vi "Check Mode Delay Update.vi"(7 "TreeControl in":refnum<vi>, 8 "Analog Changed":bool=TRUE, 9 "New Num":i32, 10 "Settings In in":T1, 11 "Tree Data in":cluster{"Tag":string[], "Settings":T3[]} {"Settings"."Data Type" items=["Tree Parent"=-1, "Numeric"=0, "String"=1, "Boolean"=2, "Enum"=3]}) -> (3 "Tree Data out":cluster{"Tag":string[], "Settings":T3[]} {"Settings"."Data Type" items=["Tree Parent"=-1, "Numeric"=0, "String"=1, "Boolean"=2, "Enum"=3]})   [LabVIEW 2024, in "Sequencer with Output Values.lvlib" / "Sequencer with Output Values.lvclass"]
uses:
  Sequencer with Output Values.lvclass
  Tree Item Settings.ctl
  Data Type.ctl
  Params.ctl
  Step Settings.ctl
  Global Tree Data.vi
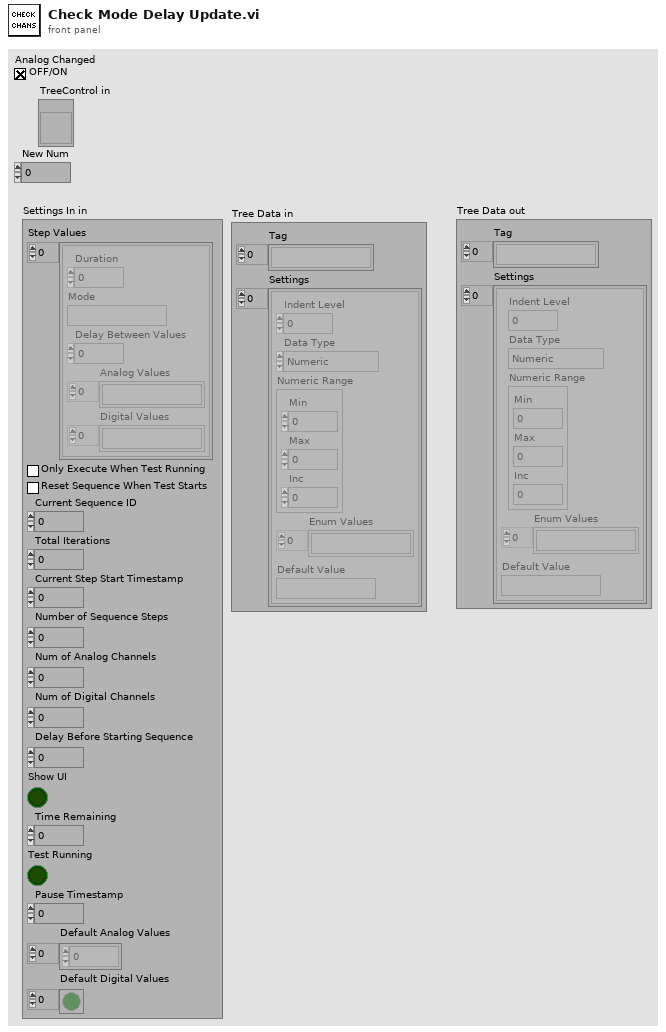
[diagram p1: front panel]
types:
  T1 = typedef "Sequencer with Output Values.lvlib/Sequencer with Output Values.lvclass/Params.ctl" = cluster{"Step Values":T2[], "Only Execute When Test Running":bool, "Reset Sequence When Test Starts":bool, "Current Sequence ID":u32, "Total Iterations":u32, "Current Step Start Timestamp":dbl, "Number of Sequence Steps":i32, "Num of Analog Channels":i32, "Num of Digital Channels":i32, "Delay Before Starting Sequence":dbl, "Show UI":bool, "Time Remaining":dbl, "Test Running":bool, "Pause Timestamp":dbl, "Default Analog Values":dbl[], "Default Digital Values":bool[]}
  T2 = typedef "Sequencer with Output Values.lvlib/Sequencer with Output Values.lvclass/Step Settings.ctl" = cluster{"Duration":dbl, "Mode":string, "Delay Between Values":dbl, "Analog Values":string[], "Digital Values":string[]}
  T3 = typedef "Sequencer with Output Values.lvlib/Sequencer with Output Values.lvclass/Tree Item Settings.ctl" = cluster{"Indent Level":i32, "Data Type":T4, "Numeric Range":cluster{"Min":dbl, "Max":dbl, "Inc":dbl}, "Enum Values":string[], "Default Value":string}
  T4 = typedef "Sequencer with Output Values.lvlib/Sequencer with Output Values.lvclass/Data Type.ctl" = i16
  T5 = cluster{"Tags Out":string[], "Settings Out":T3[]}
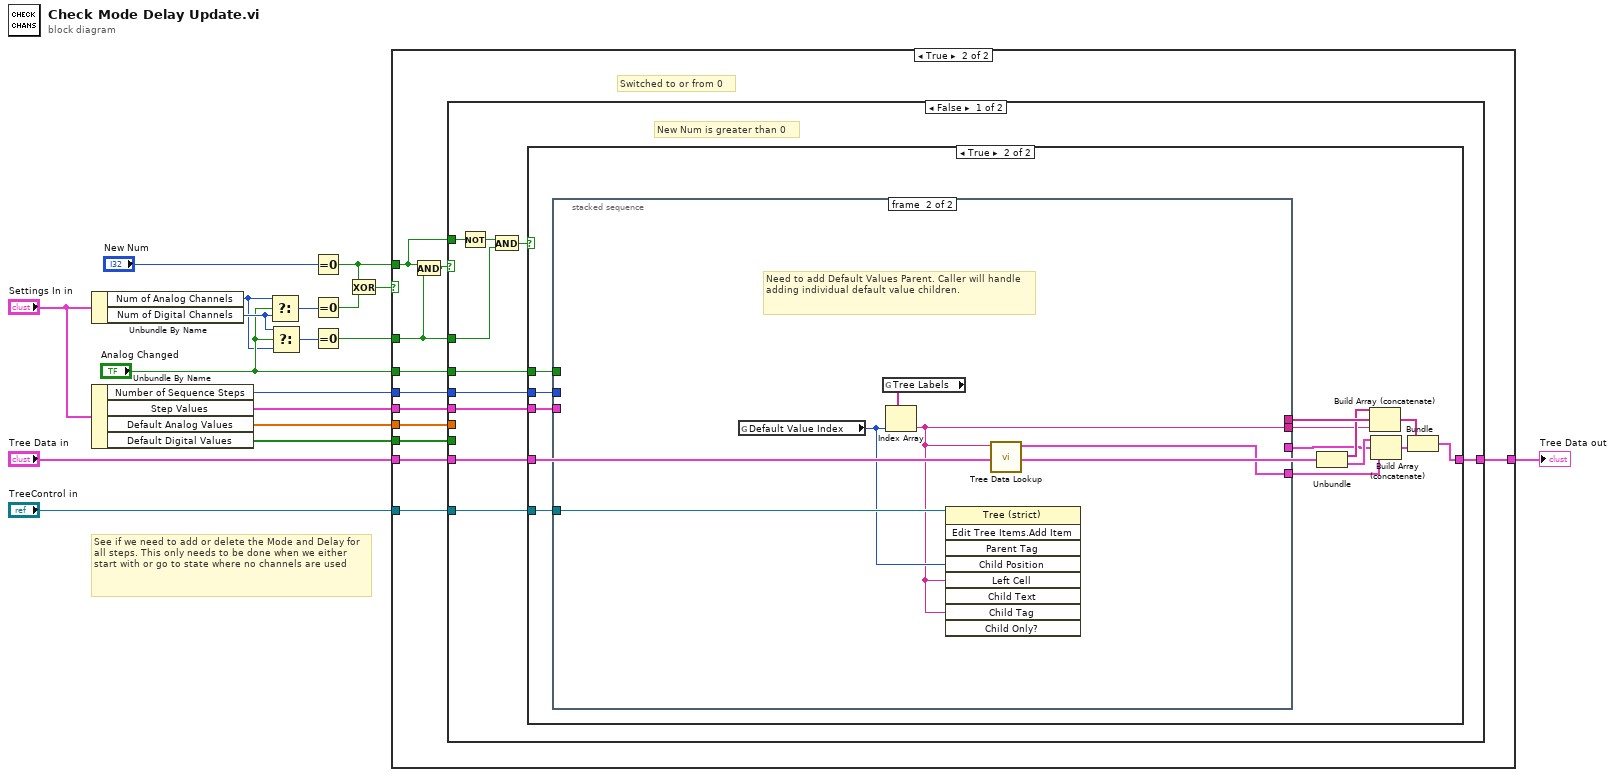
[diagram p0: block diagram]
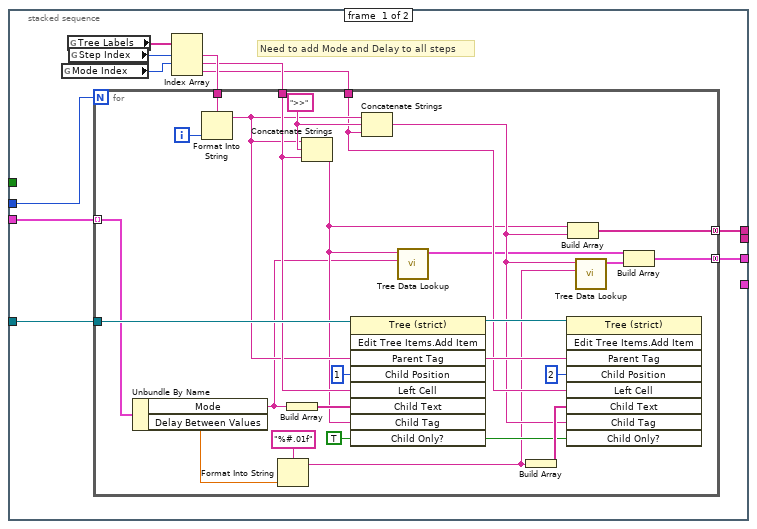
[diagram p4: hidden frame]
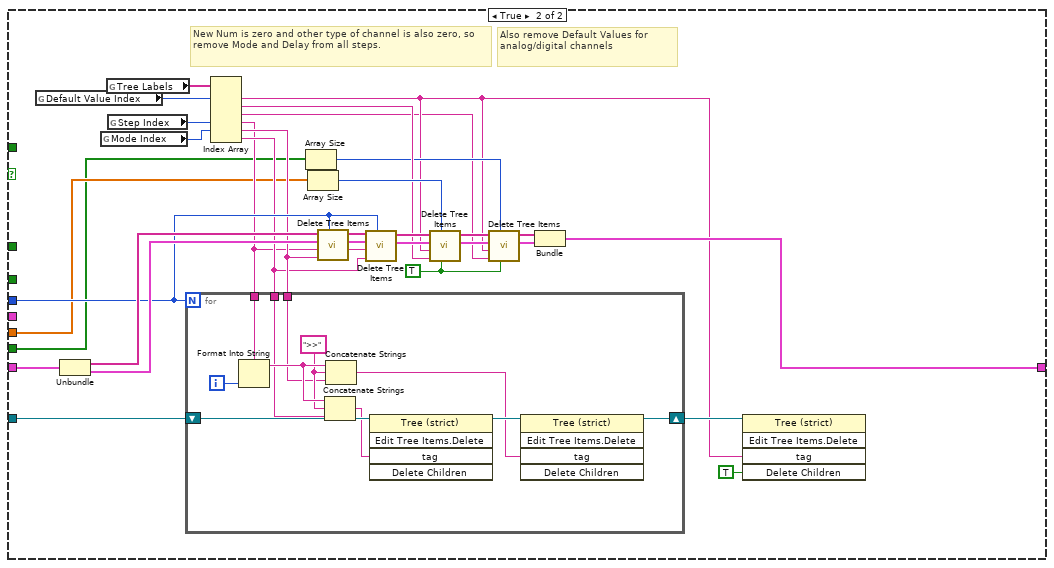
[diagram p5: hidden frame]
diagram:
  # "See if we need to add or delete the Mode and Delay for all steps. This only needs to be done when we either start with or go to state where no channels are used"
  n1 = Unbundle By Name("Settings In in") -> ("Num of Analog Channels"=w4:i32, "Num of Digital Channels"=w14:i32)
  n2 = Unbundle By Name("Settings In in") -> ("Number of Sequence Steps"=w8:i32, "Step Values"=w5:T2[], "Default Analog Values"=w3:dbl[], "Default Digital Values"=w2:bool[])
  n3 = Select(t=w4, s="Analog Changed", f=w14) -> (s? t:f=w18:i32)
  n4 = Select(t=w14, s="Analog Changed", f=w4) -> (s? t:f=w13:i32)
  n5 = Equal To 0?(x="New Num") -> (x = 0?=w15:bool)
  n6 = Equal To 0?(x=w18) -> (x = 0?=w17:bool)
  n7 = Equal To 0?(x=w13) -> (x = 0?=w12:bool)
  n8 = Exclusive Or(1:w17, 2:w15) -> (0:w16:bool)
  n9 = case shown="True" w16 {
    tunnel: w15 -> [_ w25]
    tunnel: w12 -> [_ w24]
    tunnel: "TreeControl in" -> [_ w29]
    tunnel: "Tree Data in" -> [w19 w28]
    tunnel: w8 -> [_ w27]
    tunnel: [w19 w26] -> w7
    tunnel: "Analog Changed" -> [_ w23]
    tunnel: w5 -> [_ w22]
    tunnel: w3 -> [_ w21]
    tunnel: w2 -> [_ w20]
    frame False {
      # "Change didn't affect if we should or should not display Mode and Delay"
    }
    frame True {
      # "Switched to or from 0"
      n10 = And(x=w25, y=w24) -> (x .and. y?=w30:bool)
      n11 = case shown="False" w30 {
        tunnel: w29 -> [w33 w123]
        tunnel: w28 -> [w36 w122]
        tunnel: w27 -> [w32 w114]
        tunnel: [w35 w121] -> w26
        tunnel: w25 -> [w40 _]
        tunnel: w24 -> [w38 _]
        tunnel: w23 -> [w34 _]
        tunnel: w22 -> [w31 _]
        tunnel: w21 -> [_ w108]
        tunnel: w20 -> [_ w102]
        frame False {
          # "New Num is greater than 0"
          n12 = Not(x=w40) -> (.not. x?=w39:bool)
          n13 = And(x=w39, y=w38) -> (x .and. y?=w37:bool)
          n14 = case shown="True" w37 {
            tunnel: w36 -> [w41 w52]
            tunnel: [w41 w45] -> w35
            tunnel: w34 -> [_ w44]
            tunnel: w33 -> [_ w55]
            tunnel: w32 -> [_ w54]
            tunnel: w31 -> [_ w53]
            frame False {
            }
            frame True {
              n15 = stacked-sequence {
                tunnel: w55 -> [w66 w94]
                tunnel: w54 -> [w62 _]
                tunnel: w53 -> [w59 _]
                tunnel: [w57 _] -> w51
                tunnel: [w56 _] -> w48
                tunnel: w44 -> [_ _]
                tunnel: [_ w92] -> w43
                tunnel: [_ w91] -> w42
                frame #0 {
                  # "Need to add Mode and Delay to all steps"
                  n16 = global read "Global Tree Data.vi" "Mode Index"() -> (w63:i32)
                  n17 = global read "Global Tree Data.vi" "Tree Labels"() -> (w65:string[])
                  n18 = global read "Global Tree Data.vi" "Step Index"() -> (w64:i32)
                  n19 = Index Array(array=w65, index #1=w64, index #2=w63) -> (element #1=w61:string, element #2=w60:string, element #3=w58:string)  [unwired: 1 in]
                  n20 = for {
                    N: w62 -> [_]
                    tunnel: w66 -> [w90]
                    tunnel: w61 -> [w89]
                    tunnel: w60 -> [w87]
                    tunnel: w59 -> [w85] mode=indexing
                    tunnel: w58 -> [w79]
                    tunnel: [w73] -> w57 mode=concatenating
                    tunnel: [w67] -> w56 mode=concatenating
                    i -> [w88]
                    w75 = TRUE ("Child Only?")
                    w82 = ">>" ("string")
                    n21 = Unbundle By Name(w85) -> ("Mode"=w69:string, "Delay Between Values"=w78:dbl)
                    n22 = Format Into String(format string=w89, w88) -> (resulting string=w81:string)  [unwired: 2 in, 1 out]
                    n23 = Format Into String(format string="%#.01f", w78) -> (resulting string=w72:string)  [unwired: 2 in, 1 out]
                    n24 = Build Array(w69) -> (w84:string[])
                    n25 = Concatenate Strings(w81, w82, w87) -> (w70:string)
                    n26 = invoke class="Tree (strict)" method="Edit Tree Items.Add Item"(reference=w90, "Parent Tag"=w81, "Child Position"=1, "Left Cell"=w87, "Child Text"=w84, "Child Tag"=w70, "Child Only?"=w75) -> (reference out=w83:refnum<vi>)  [unwired: 2 in, 8 out]
                    n27 = Concatenate Strings(w81, w82, w79) -> (w74:string)
                    n28 = call "Tree Data Lookup.vi"("Value"=w69, "Key"=w70) -> ("Tree Data"=w68:T3)  [unwired: 9 in]
                    n29 = Build Array(w72) -> (w76:string[])
                    n30 = invoke class="Tree (strict)" method="Edit Tree Items.Add Item"(reference=w83, "Parent Tag"=w81, "Child Position"=2, "Left Cell"=w79, "Child Text"=w76, "Child Tag"=w74, "Child Only?"=w75) -> ()  [unwired: 2 in, 9 out]
                    n31 = Build Array(w70, w74) -> (w73:string[])
                    n32 = call "Tree Data Lookup.vi"("Value"=w72, "Key"=w74) -> ("Tree Data"=w71:T3)  [unwired: 9 in]
                    n33 = Build Array(w68, w71) -> (w67:T3[])
                  }
                }
                frame #1 {
                  # "Need to add Default Values Parent. Caller will handle adding individual default value children."
                  n34 = global read "Global Tree Data.vi" "Default Value Index"() -> (w93:i32)
                  n35 = global read "Global Tree Data.vi" "Tree Labels"() -> (w95:string[])
                  n36 = Index Array(array=w95, index=w93) -> (element=w92:string)
                  n37 = invoke class="Tree (strict)" method="Edit Tree Items.Add Item"(reference=w94, "Child Position"=w93, "Left Cell"=w92, "Child Tag"=w92) -> ()  [unwired: 5 in, 9 out]
                  n38 = call "Tree Data Lookup.vi"("Key"=w92) -> ("Tree Data"=w91:T3)  [unwired: 10 in]
                }
              }
              n39 = Unbundle(w52) -> ("Tag"=w50:string[], "Settings"=w49:T3[])
              n40 = Build Array (concatenate)(w50, w51, w43) -> (w47:string[])
              n41 = Build Array (concatenate)(w49, w48, w42) -> (w46:T3[])
              n42 = Bundle(w47, w46) -> (w45:cluster{string[], T3[]})  [unwired: 1 in]
            }
          }
        }
        frame True {
          w98 = TRUE ("Try to delete parent as well")
          # "Also remove Default Values for analog/digital channels"
          # "New Num is zero and other type of channel is also zero, so remove Mode and Delay from all steps."
          n43 = global read "Global Tree Data.vi" "Default Value Index"() -> (w106:i32)
          n44 = Unbundle(w122) -> ("Tag"=w118:string[], "Settings"=w117:T3[])
          n45 = global read "Global Tree Data.vi" "Mode Index"() -> (w124:i32)
          n46 = global read "Global Tree Data.vi" "Tree Labels"() -> (w126:string[])
          n47 = global read "Global Tree Data.vi" "Step Index"() -> (w125:i32)
          n48 = Index Array(array=w126, index #1=w106, index #4=w125, index #5=w124) -> (element #1=w100:string, element #2=w105:string, element #3=w99:string, element #4=w111:string, element #5=w113:string, element #6=w112:string)  [unwired: 3 in]
          n49 = for {
            N: w114 -> [_]
            tunnel: w111 -> [w137]
            tunnel: w113 -> [w132]
            tunnel: w112 -> [w131]
            shift-right: [w127] -> w120
            shift-left: w123 -> [w135]
            i -> [w136]
            w133 = ">>" ("string")
            n50 = Format Into String(format string=w137, w136) -> (resulting string=w134:string)  [unwired: 2 in, 1 out]
            n51 = Concatenate Strings(w134, w133, w131) -> (w129:string)
            n52 = Concatenate Strings(w134, w133, w132) -> (w128:string)
            n53 = invoke class="Tree (strict)" method="Edit Tree Items.Delete"(reference=w135, "tag"=w129) -> (reference out=w130:refnum<vi>)  [unwired: 3 in, 4 out]
            n54 = invoke class="Tree (strict)" method="Edit Tree Items.Delete"(reference=w130, "tag"=w128) -> (reference out=w127:refnum<vi>)  [unwired: 3 in, 4 out]
          }
          n55 = Array Size(array=w102) -> (size(s)=w101:i32)
          n56 = Array Size(array=w108) -> (size(s)=w107:i32)
          n57 = call "Delete Tree Items.vi"("Num of Items to Remove"=w114, "Child String"=w113, "Parent String"=w111, "Settings In"=w117, "Tags In"=w118) -> ("Settings Out"=w115:T3[], "Tags Out"=w116:string[])  [unwired: 5 in]
          n58 = call "Delete Tree Items.vi"("Num of Items to Remove"=w114, "Child String"=w112, "Parent String"=w111, "Settings In"=w115, "Tags In"=w116) -> ("Settings Out"=w109:T3[], "Tags Out"=w110:string[])  [unwired: 5 in]
          n59 = call "Delete Tree Items.vi"("Try to delete parent as well"=w98, "Num of Items to Remove"=w107, "Child String"=w105, "Parent String"=w100, "Settings In"=w109, "Tags In"=w110) -> ("Settings Out"=w103:T3[], "Tags Out"=w104:string[])  [unwired: 4 in]
          n60 = call "Delete Tree Items.vi"("Try to delete parent as well"=w98, "Num of Items to Remove"=w101, "Child String"=w99, "Parent String"=w100, "Settings In"=w103, "Tags In"=w104) -> ("Settings Out"=w96:T3[], "Tags Out"=w97:string[])  [unwired: 4 in]
          n61 = Bundle("Tags Out"=w97, "Settings Out"=w96) -> (w121:T5)  [unwired: 1 in]
          n62 = invoke class="Tree (strict)" method="Edit Tree Items.Delete"(reference=w120, "tag"=w100, "Delete Children"=TRUE ("Delete Children?")) -> ()  [unwired: 2 in, 5 out]
        }
      }
    }
  }
  "Tree Data out" <- w7
